vi "Teleop.vi"(10 "Match Info":T1={"Autonomous Elapsed Seconds"=0.0, "TeleOp Elapsed Seconds"=0.0, "Disabled Elapsed Seconds"=0.0, "Visited Autonomous"=FALSE, "Visited TeleOp"=FALSE, "Visited Disabled"=FALSE, "Autonomous Settings"={"Autonomous Style"=enum."Independent", "VI Refnum"=refnum}}, 11 "Call Context":T2) -> ()   [LabVIEW 2014]
doc: "This VI is called for each TeleOp packet received from the DS where the robot is not disabled. It is often used to read from the joysticks and update I/O or to update setpoints for timed control loops. It should complete and return within 20 milliseconds or it may miss DS packets."
uses:
  <vilib>/Rock Robotics/WPI/DriverStation/WPI_DriverStationDerivedRobotMode.ctl
  <vilib>/Rock Robotics/WPI/DriverStation/WPI_DriverStationMatch Info.ctl
  <vilib>/Rock Robotics/WPI/Joystick/WPI_JoystickGetSetRefNum.vi
  <vilib>/Rock Robotics/Network Tables/SD Write Boolean Array.vi
  <vilib>/Rock Robotics/Network Tables/SD Write Numeric Array.vi
  <vilib>/Rock Robotics/Network Tables/SD Read Boolean.vi
  <vilib>/Rock Robotics/Network Tables/SD Read Number.vi
  Support Files/Global Data!!!.vi
panel:
  out "Sample Slider 0":dbl(slide) scale=0.0..5.0
  out "Sample Boolean 1":bool
  out "Sample Boolean 0":bool
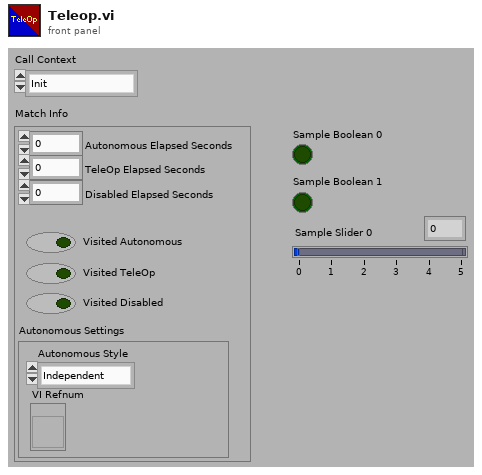
[diagram p1: front panel]
types:
  T1 = typedef "WPI_DriverStationMatch Info.ctl" = cluster{"Autonomous Elapsed Seconds":dbl, "TeleOp Elapsed Seconds":dbl, "Disabled Elapsed Seconds":dbl, "Visited Autonomous":bool, "Visited TeleOp":bool, "Visited Disabled":bool, "Autonomous Settings":cluster{"Autonomous Style":enum16{"Iterative", "Independent"}, "VI Refnum":refnum<vi>}}
  T2 = typedef "WPI_DriverStationDerivedRobotMode.ctl" = enum16{"Init", "Execute", "Stop"}
  T3 = typedef "WPI_JoystickDevRef.ctl" = cluster{"Device":T4}
  T4 = typedef "WPI_JoystickDeviceEnum.ctl" = enum16{"USB 0", "USB 1", "USB 2", "USB 3", "USB 4", "USB 5"}
  T5 = cluster{"Axes[0]":dbl, "Axes[1]":dbl, "Axes[2]":dbl, "Axes[3]":dbl, "Axes[4]":dbl, "Axes[5]":dbl, "Axes[6]":dbl, "Axes[7]":dbl, "Axes[8]":dbl}
  T6 = cluster{"Buttons[0]":bool, "Buttons[1]":bool, "Buttons[2]":bool, "Buttons[3]":bool, "Buttons[4]":bool, "Buttons[5]":bool, "Buttons[6]":bool, "Buttons[7]":bool, "Buttons[8]":bool}
  T7 = cluster{"POVs[0]":i16, "POVs[1]":i16, "POVs[2]":i16, "POVs[3]":i16, "POVs[4]":i16, "POVs[5]":i16, "POVs[6]":i16, "POVs[7]":i16, "POVs[8]":i16}
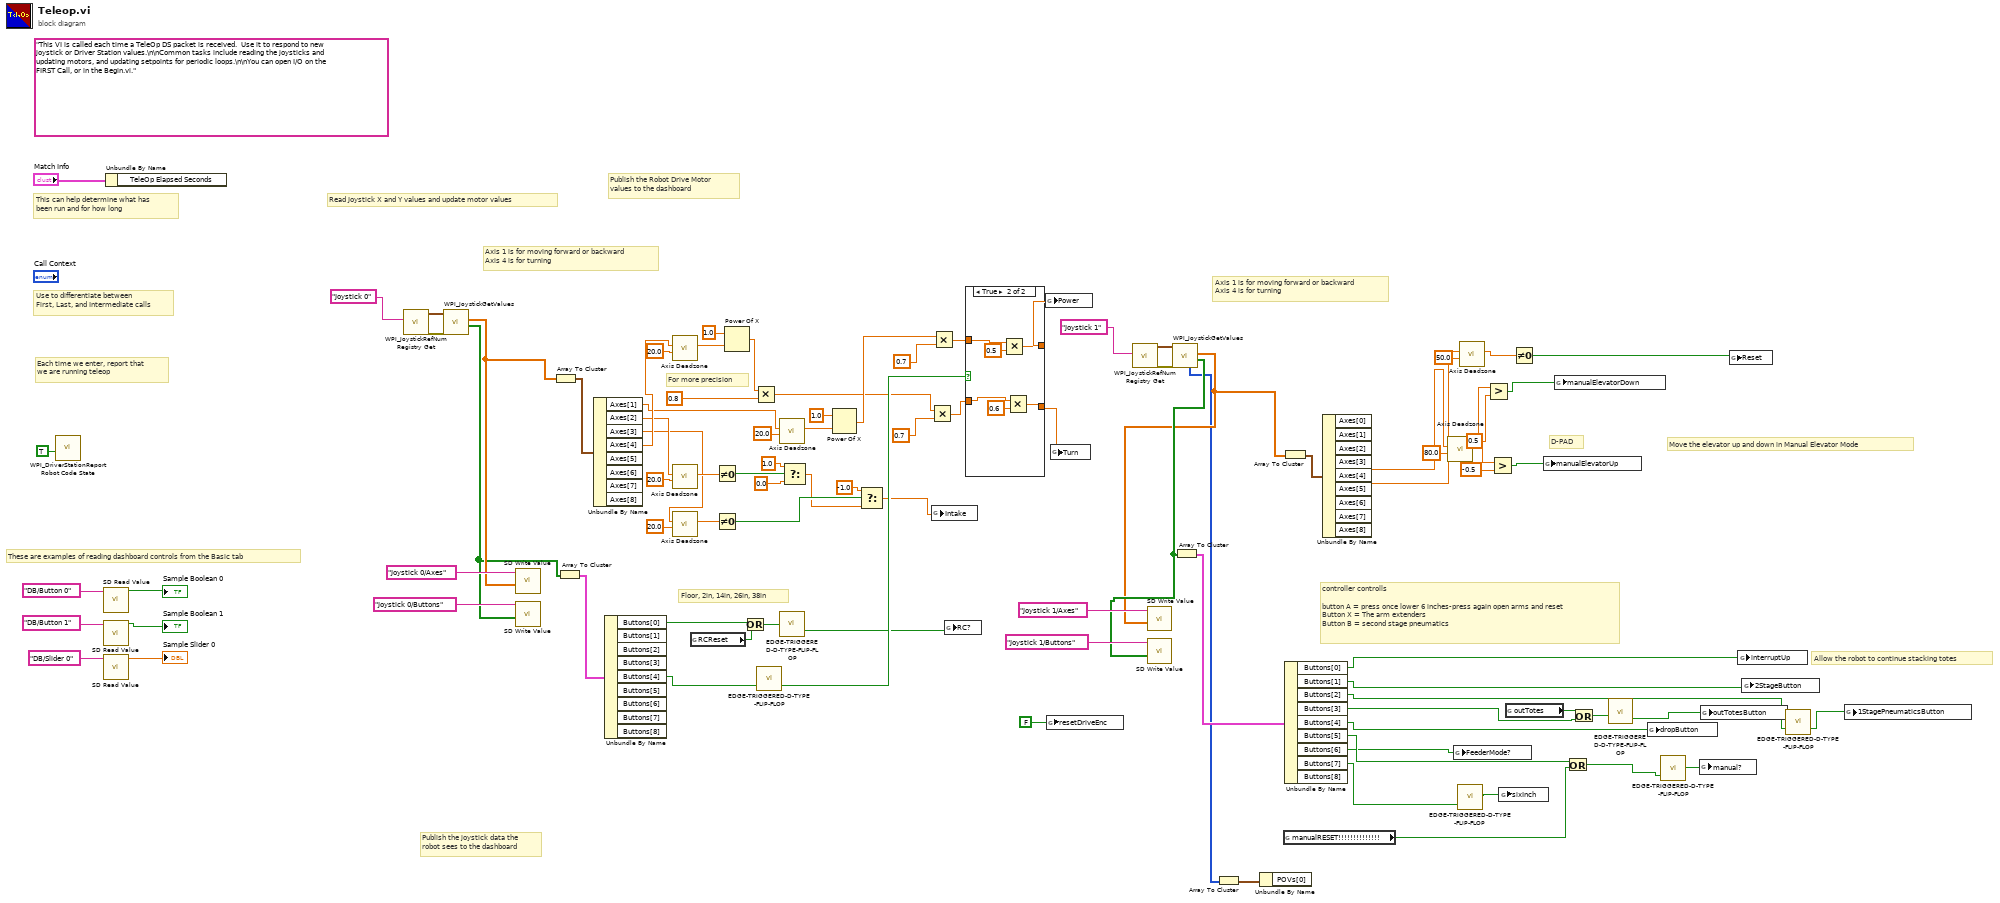
[diagram p0: block diagram]
diagram:
  (unwired) "This VI is called each time a TeleOp DS packet is received.  Use it to respond to new joystick or Driver Station values.\n\nCommon tasks include reading the joysticks and updating motors, and updating setpoints for periodic loops.\n\nYou can open I/O on the FIRST Call, or in the Begin.vi."
  # "For more precision"
  # "D-PAD"
  # "Allow the robot to continue stacking totes"
  # "Move the elevator up and down in Manual Elevator Mode"
  # "Floor, 2in, 14in, 26in, 38in"
  # "controller controlls\n\nbutton A = press once lower 6 inches-press again open arms and reset\nButton X = The arm extenders\nButton B = second stage pneumatics"
  # "Axis 1 is for moving forward or backward\nAxis 4 is for turning"
  # "Axis 1 is for moving forward or backward\nAxis 4 is for turning"
  # "These are examples of reading dashboard controls from the Basic tab"
  # "Publish the Robot Drive Motor\nvalues to the dashboard"
  # "Publish the joystick data the\nrobot sees to the dashboard"
  # "Each time we enter, report that\nwe are running teleop"
  # "Use to differentiate between\nFirst, Last, and Intermediate calls"
  # "This can help determine what has\nbeen run and for how long"
  # "Read Joystick X and Y values and update motor values"
  n1 = call <vilib>:"WPI_DriverStationReport Robot Code State.vi"("TeleOp"=TRUE ("Autonomous")) -> ()  [unwired: 10 in, 1 out]
  n2 = call-poly <vilib>:"SD Read Value.vi"("Name"="DB/Button 0" ("refnum name")) -> ("Boolean"=→"Sample Boolean 0":bool)  [unwired: 8 in, 2 out]
  n3 = call-poly <vilib>:"SD Read Value.vi"("Name"="DB/Button 1" ("refnum name")) -> ("Boolean"=→"Sample Boolean 1":bool)  [unwired: 8 in, 2 out]
  n4 = call-poly <vilib>:"SD Read Value.vi"("Name"="DB/Slider 0" ("refnum name")) -> ("Numeric"=→"Sample Slider 0":dbl)  [unwired: 8 in, 2 out]
  n5 = Unbundle By Name("Match Info") -> ()  [unwired: 1 out]
  n6 = call <vilib>:"WPI_JoystickRefNum Registry Get.vi"("refnum name"="Joystick 0") -> ("error out"=w81:errorcluster, "JoystickDevRef"=w91:T3)  [unwired: 1 in, 8 out]
  n7 = call <vilib>:"WPI_JoystickGetValues.vi"("error in (no error)"=w81, "JoystickDevRef"=w91) -> ("Buttons"=w78:bool[], "Axes"=w80:dbl[])  [unwired: 5 in, 3 out]
  n8 = call-poly <vilib>:"SD Write Value.vi"("Numeric Array"=w80, "Name"="Joystick 0/Axes") -> ()  [unwired: 8 in, 2 out]
  n9 = call-poly <vilib>:"SD Write Value.vi"("Boolean Array"=w78, "Name"="Joystick 0/Buttons") -> ()  [unwired: 8 in, 2 out]
  n10 = Array To Cluster(array=w80) -> (cluster=w79:T5)
  n11 = Array To Cluster(array=w78) -> (cluster=w77:T6)
  n12 = Unbundle By Name(w79) -> ("Axes[1]"=w35:dbl, "Axes[2]"=w10:dbl, "Axes[3]"=w9:dbl, "Axes[4]"=w71:dbl)  [unwired: 4 out]
  n13 = Unbundle By Name(w77) -> ("Buttons[0]"=w20:bool, "Buttons[4]"=w28:bool)  [unwired: 7 out]
  n14 = call "Axis Deadzone.vi"("% Deadzone (Default 5%)"=20.0, "Axis Input"=w71) -> ("Output With Deadzone"=w33:dbl)  [unwired: 9 in]
  n15 = call "Axis Deadzone.vi"("% Deadzone (Default 5%)"=20.0, "Axis Input"=w10) -> ("Output With Deadzone"=w15:dbl)  [unwired: 9 in]
  n16 = call "Axis Deadzone.vi"("% Deadzone (Default 5%)"=20.0, "Axis Input"=w9) -> ("Output With Deadzone"=w11:dbl)  [unwired: 9 in]
  n17 = global read "Global Data!!!.vi" "RCReset"() -> (w19:bool)
  n18 = Not Equal To 0?(x=w15) -> (x != 0?=w8:bool)
  n19 = Not Equal To 0?(x=w11) -> (x != 0?=w7:bool)
  n20 = Power Of X(1:w33, 2:1.0 ("x")) -> (0:w30:dbl)
  n21 = Or(x=w20, y=w19) -> (x .or. y?=w21:bool)
  n22 = Multiply(x=w30, y=0.8) -> (x*y=w2:dbl)
  n23 = call "EDGE-TRIGGERED-D-TYPE-FLIP-FLOP.vi"("WRITE"=w28) -> ("Q-bar"=w24:bool)  [unwired: 2 in]
  n24 = call "Axis Deadzone.vi"("% Deadzone (Default 5%)"=20.0, "Axis Input"=w35) -> ("Output With Deadzone"=w36:dbl)  [unwired: 9 in]
  n25 = call "EDGE-TRIGGERED-D-TYPE-FLIP-FLOP.vi"("WRITE"=w21) -> ("Q-bar"=w22:bool)  [unwired: 2 in]
  n26 = Select(t=1.0, s=w8, f=0.0) -> (s? t:f=w6:dbl)
  n27 = Power Of X(1:w36, 2:1.0 ("x")) -> (0:w31:dbl)
  n28 = Select(t=-1.0, s=w7, f=w6) -> (s? t:f=w5:dbl)
  n29 = Multiply(x=w2, y=0.7) -> (x*y=w3:dbl)
  n30 = Multiply(x=w31, y=0.7) -> (x*y=w26:dbl)
  n31 = global write "Global Data!!!.vi" "Intake"(w5) -> ()
  n32 = global write "Global Data!!!.vi" "RC?"(w22) -> ()
  n33 = case shown="True" w24 {
    tunnel: [w95 w100] -> w27
    tunnel: w26 -> [w95 w101]
    tunnel: w3 -> [w94 w97]
    tunnel: [w94 w96] -> w25
    frame False {
    }
    frame True {
      n34 = Multiply(x=w101, y=0.5) -> (x*y=w100:dbl)
      n35 = Multiply(x=w97, y=0.6) -> (x*y=w96:dbl)
    }
  }
  n36 = global write "Global Data!!!.vi" "Power"(w27) -> ()
  n37 = global write "Global Data!!!.vi" "resetDriveEnc"(FALSE ("resetDriveEnc")) -> ()
  n38 = global write "Global Data!!!.vi" "Turn"(w25) -> ()
  n39 = call <vilib>:"WPI_JoystickRefNum Registry Get.vi"("refnum name"="Joystick 1") -> ("error out"=w75:errorcluster, "JoystickDevRef"=w74:T3)  [unwired: 1 in, 8 out]
  n40 = call <vilib>:"WPI_JoystickGetValues.vi"("error in (no error)"=w75, "JoystickDevRef"=w74) -> ("Buttons"=w66:bool[], "Axes"=w65:dbl[], "POVs"=w59:i16[])  [unwired: 5 in, 2 out]
  n41 = call-poly <vilib>:"SD Write Value.vi"("Numeric Array"=w65, "Name"="Joystick 1/Axes") -> ()  [unwired: 8 in, 2 out]
  n42 = call-poly <vilib>:"SD Write Value.vi"("Boolean Array"=w66, "Name"="Joystick 1/Buttons") -> ()  [unwired: 8 in, 2 out]
  n43 = Array To Cluster(array=w66) -> (cluster=w69:T6)
  n44 = Array To Cluster(array=w59) -> (cluster=w58:T7)
  n45 = Unbundle By Name(w58) -> ()  [unwired: 1 out]
  n46 = Array To Cluster(array=w65) -> (cluster=w76:T5)
  n47 = global read "Global Data!!!.vi" "manualRESET!!!!!!!!!!!!!!"() -> (w55:bool)
  n48 = Unbundle By Name(w69) -> ("Buttons[0]"=w53:bool, "Buttons[1]"=w39:bool, "Buttons[2]"=w50:bool, "Buttons[3]"=w48:bool, "Buttons[4]"=w52:bool, "Buttons[5]"=w54:bool, "Buttons[6]"=w18:bool, "Buttons[7]"=w51:bool)  [unwired: 1 out]
  n49 = Unbundle By Name(w76) -> ("Axes[1]"=w38:dbl, "Axes[2]"=w63:dbl)  [unwired: 7 out]
  n50 = call "Axis Deadzone.vi"("% Deadzone (Default 5%)"=80.0, "Axis Input"=w38) -> ("Output With Deadzone"=w44:dbl)  [unwired: 9 in]
  n51 = global write "Global Data!!!.vi" "FeederMode?"(w18) -> ()
  n52 = call "EDGE-TRIGGERED-D-TYPE-FLIP-FLOP.vi"("WRITE"=w51) -> ("Q-bar"=w56:bool)  [unwired: 2 in]
  n53 = call "Axis Deadzone.vi"("% Deadzone (Default 5%)"=50.0, "Axis Input"=w63) -> ("Output With Deadzone"=w61:dbl)  [unwired: 9 in]
  n54 = Greater?(x=w44, y=0.5) -> (0:w43:bool)
  n55 = Greater?(x=w44, y=-0.5) -> (0:w42:bool)
  n56 = global write "Global Data!!!.vi" "sixInch"(w56) -> ()
  n57 = global read "Global Data!!!.vi" "outTotes"() -> (w47:bool)
  n58 = Not Equal To 0?(x=w61) -> (x != 0?=w60:bool)
  n59 = global write "Global Data!!!.vi" "manualElevatorUp"(w42) -> ()
  n60 = global write "Global Data!!!.vi" "manualElevatorDown"(w43) -> ()
  n61 = Or(x=w54, y=w55) -> (x .or. y?=w23:bool)
  n62 = Or(x=w47, y=w48) -> (x .or. y?=w49:bool)
  n63 = call "EDGE-TRIGGERED-D-TYPE-FLIP-FLOP.vi"("WRITE"=w49) -> ("Q-bar"=w1:bool)  [unwired: 2 in]
  n64 = global write "Global Data!!!.vi" "dropButton"(w52) -> ()
  n65 = call "EDGE-TRIGGERED-D-TYPE-FLIP-FLOP.vi"("WRITE"=w23) -> ("Q-bar"=w64:bool)  [unwired: 2 in]
  n66 = global write "Global Data!!!.vi" "manual?"(w64) -> ()
  n67 = global write "Global Data!!!.vi" "outTotesButton"(w1) -> ()
  n68 = global write "Global Data!!!.vi" "Reset"(w60) -> ()
  n69 = global write "Global Data!!!.vi" "interruptUp"(w53) -> ()
  n70 = global write "Global Data!!!.vi" "2StageButton"(w39) -> ()
  n71 = call "EDGE-TRIGGERED-D-TYPE-FLIP-FLOP.vi"("WRITE"=w50) -> ("Q-bar"=w57:bool)  [unwired: 2 in]
  n72 = global write "Global Data!!!.vi" "1StagePneumaticsButton"(w57) -> ()
